vi "Close Directed Graph Map.vi"(8 "error in (no error)":errorcluster, 11 "map reference in":refnum<data-value>) -> (0 "error out":errorcluster)   [LabVIEW 2017, in "NI_Robotics_DirectedGraphWorldMap.lvclass"]
doc: "Closes an open reference to a directed graph map object."
uses:
  <vilib>/robotics/Navigation/shared/WorldMap/DirectedGraphWorldMap/NI_Robotics_DirectedGraphWorldMap.lvclass
  <vilib>/robotics/Navigation/shared/WorldMap/DirectedGraphWorldMap/NI_Robotics_DirectedGraphWorldMap.lvclass/NI_Robotics_DirectedGraphWorldMap.ctl
  <vilib>/robotics/Navigation/shared/MapNode/DirectedGraphMapNode/NI_Robotics_DirectedGraphMapNode.lvclass
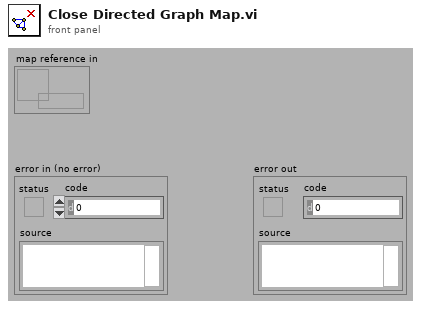
[diagram p1: front panel]
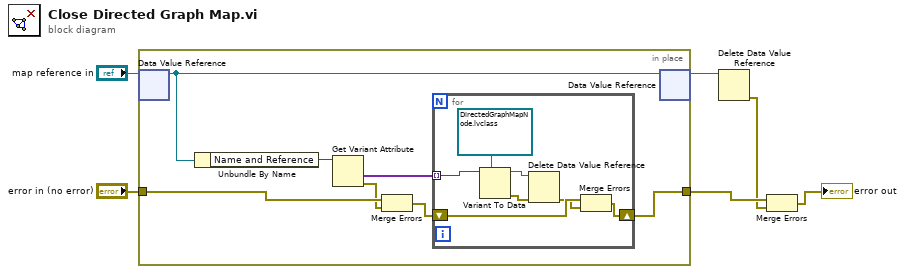
[diagram p0: block diagram]
diagram:
  n1 = in-place {
    in-place-border: "error in (no error)" -> [w9]
    in-place-border: [w10] -> w3
    n2 = in-place-dvr #1("map reference in") -> (w13:refnum<class "NI_Robotics_DirectedGraphWorldMap.lvclass">)  [unwired: 1 out]
    n3 = Unbundle By Name(w13) -> ("Name and Reference"=w12:variant)
    n4 = Get Variant Attribute(Variant=w12) -> (values=w11:variant[], error out=w8:errorcluster)  [unwired: 3 in, 2 out]
    n5 = Merge Errors(w9, w8) -> (w7:errorcluster)
    n6 = for {
      tunnel: w11 -> [w19] mode=indexing
      shift-right: [w14] -> w10
      shift-left: w7 -> [w16]
      n7 = Variant To Data(type=refnum<data-value> refnum ("Node ref"), Variant=w19) -> (data=w17:refnum<data-value>, error out=w20:errorcluster)  [unwired: 1 in]
      n8 = Delete Data Value Reference(data value reference=w17, error in=w20) -> (error out=w15:errorcluster)  [unwired: 1 out]
      n9 = Merge Errors(w16, w15) -> (w14:errorcluster)
    }
    n10 = in-place-dvr #1(w13) -> (w4:refnum<data-value>)  [unwired: 1 out]
  }
  n11 = Delete Data Value Reference(data value reference=w4) -> (error out=w2:errorcluster)  [unwired: 1 in, 1 out]
  n12 = Merge Errors(w3, w2) -> (→"error out":errorcluster)
